vi "Get Possible Connections for Endpoint.vi"(8 "error in (no error)":errorcluster, 10 "Endpoint":string, 11 "Hardware Ref in":T1 format="%.0x") -> (0 "error out":errorcluster, 2 "Possible Connections":string[](array[string]), 3 "Hardware Ref out":T1 format="%.0x")   [LabVIEW 2020, in "Routing and Faulting Hardware API.lvlib"]
uses:
  Routing and Faulting Hardware API.lvlib
  <vilib>/NI VeriStand/Custom Device API/Custom Device Item Ref.ctl
  NationalInstruments.VeriStand.SystemDefinitionAPI
  Routing and Faulting Hardware API Constants.vi
  <vilib>/NI VeriStand/Custom Device API/Custom Device API.lvlib
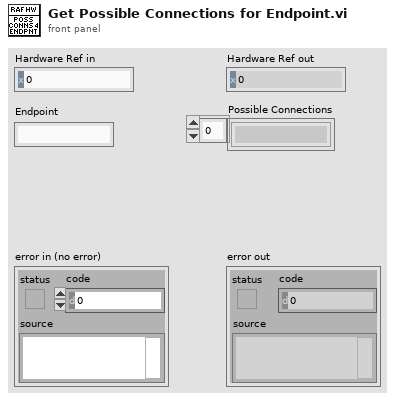
[diagram p1: front panel]
types:
  T1 = typedef "Custom Device API.lvlib/Custom Device Item Ref.ctl" = u64
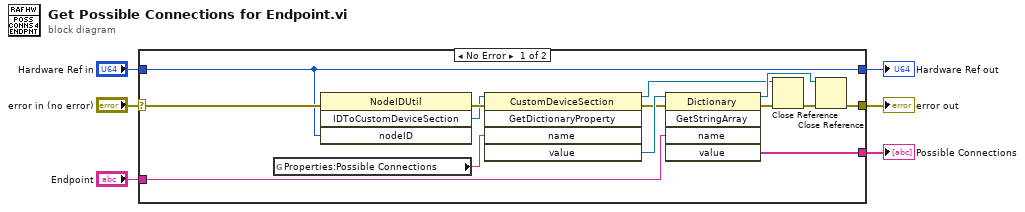
[diagram p0: block diagram]
diagram:
  n1 = case shown="No Error" "error in (no error)" {
    selector: "error in (no error)" -> [w9 w22]
    tunnel: [w19 w22] -> w6
    tunnel: "Hardware Ref in" -> [w8 w21]
    tunnel: [w8 w21] -> w3
    tunnel: [w12 _] -> w2
    tunnel: "Endpoint" -> [w7 _]
    frame No Error {
      n2 = global read "Routing and Faulting Hardware API Constants.vi" "Properties:Possible Connections"() -> (w16:string)
      n3 = invoke class="NodeIDUtil" method="IDToCustomDeviceSection"(error in=w9, "nodeID"=w8) -> (error out=w18:errorcluster, "IDToCustomDeviceSection"=w15:refnum<k24>)  [unwired: 2 in, 2 out]
      n4 = invoke class="CustomDeviceSection" method="GetDictionaryProperty"(reference=w15, error in=w18, "name"=w16) -> (reference out=w10:refnum<k24>, error out=w14:errorcluster, "value"=w17:refnum<k24>)  [unwired: 2 in, 2 out]
      n5 = invoke class="Dictionary" method="GetStringArray"(reference=w17, error in=w14, "name"=w7) -> (reference out=w11:refnum<k24>, error out=w13:errorcluster, "value"=w12:string[])  [unwired: 2 in, 2 out]
      n6 = Close Reference(reference=w10, error in (no error)=w13) -> (error out=w20:errorcluster)
      n7 = Close Reference(reference=w11, error in (no error)=w20) -> (error out=w19:errorcluster)
    }
    frame Error {
    }
  }
  "Hardware Ref out" <- w3
  "error out" <- w6
  "Possible Connections" <- w2
